vi "leds.vi"() -> ()   [LabVIEW 2018]
uses:
  <vilib>/DAQmx/read.llb/DAQmx Read (Digital 1D Bool NChan 1Samp 1Line).vi
  <vilib>/DAQmx/miscellaneous.llb/DAQmx Fill In Error Info.vi
panel:
  out "data 2":bool[](array[boolean])
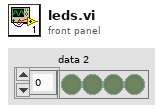
[diagram p1: front panel]
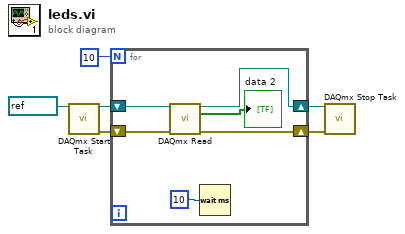
[diagram p0: block diagram]
diagram:
  n1 = call <vilib>:"DAQmx Start Task.vi"("task/channels in"=refnum<k21> "leds") -> ("task out"=w3:refnum<k21>, "error out"=w5:errorcluster)  [unwired: 13 in]
  n2 = for {
    N: 10 -> [_]
    shift-right: [w12] -> w6
    shift-left: w5 -> [w11]
    shift-right: [w10] -> w4
    shift-left: w3 -> [w9]
    n3 = call-poly <vilib>:"DAQmx Read.vi"("task/channels in"=w9, "error in"=w11) -> ("task out"=w10:refnum<k21>, "data"=→"data 2":bool[], "error out"=w12:errorcluster)  [unwired: 11 in]
    n4 = Wait (ms)(milliseconds to wait=u32 10) -> ()  [unwired: 1 out]
  }
  n5 = call <vilib>:"DAQmx Stop Task.vi"("task/channels in"=w4, "error in"=w6) -> ()  [unwired: 12 in, 2 out]
